vi "PieChart-New.vi"(6 "InitializationValue-Input":T2, 7 "Plot Cluster":T1, 8 "error in (no error)":errorcluster, 9 "Graph Refference's":T3, 10 "Zen Analytics in":refnum<class "Zen Analytics.lvclass">, 11 "Input_Data":dbl[][](array[numeric])=[[1.0, 2.0, 3.0, 4.0, 5.0, 6.0, 7.0, 8.0, 9.0, 10.0], [1.0, 2.0, 3.0, 4.0, 5.0, 6.0, 7.0, 8.0, 9.0, 10.0], [1.0, 2.0, 3.0, 4.0, 5.0, 6.0, 7.0, 8.0, 9.0, 10.0], [1.0, 2.0, 3.0, 4.0, 5.0, 6.0, 7.0, 8.0, 9.0, 10.0], [1.0, 2.0, 3.0, 4.0, 5.0, 6.0, 7.0, 8.0, 9.0, 10.0], [1.0, 2.0, 3.0, 4.0, 5.0, 6.0, 7.0, 8.0, 9.0, 10.0], [1.0, 2.0, 3.0, 4.0, 5.0, 6.0, 7.0, 8.0, 9.0, 10.0], [1.0, 2.0, 3.0, 4.0, 5.0, 6.0, 7.0, 8.0, 9.0, 10.0], [1.0, 2.0, 3.0, 4.0, 6.0, 6.0, 7.0, 8.0, 9.0, 10.0], [1.0, 2.0, 3.0, 4.0, 5.0, 6.0, 7.0, 8.0, 9.0, 10.0]]) -> (0 "error out":errorcluster, 4 "InitializationValues-Output":T2)   [LabVIEW 2019, in "Zen Analytics.lvlib" / "Zen Analytics.lvclass"]
uses:
  Zen Analytics.lvclass
  Dependency/GraphReff.ctl
  Dependency/Plot Cluster.ctl
panel:
  in  "ColorForProduction":u32[](array[colorbox])=[30476, 12845604]
  in  "ColorsForDefects":u32[](array[colorbox])=[10387, 14090395, 38587, 9764938, 14009600, 9961367, 16618491, 12294549, 16752640, 9614336, 35148, 16961, 2228, 13369599, 16740764, 12293546, 8152202, 7498315, 8229484, 8692651, 16744793, 12713794, 32960, 9005056, 7536640, 1638515, 3604546, 13107307, 16734575, 13107258, 4793150, 4934514]
types:
  T1 = typedef "Zen Analytics.lvlib/Zen Analytics.lvclass/Plot Cluster.ctl" = cluster{"Reduced 2D":dbl[][], "Start Index":i32, "No Of New Termnals":i32, "Top/Bottom":bool, "Values Inserted":i32, "Re-Initialised":bool, "Statistical params":string[][], "MeasurementInitializationData":cluster{"Measurement-ID":i32[], "Measurement Names":string[], "NominalValues":dbl[], "LSL":dbl[], "USL":dbl[], "LCL":dbl[], "UCL":dbl[]}, "MeasurementData":cluster{"Measurement ID":i32, "Measurement Name":string, "Nominal Values":dbl, "LSL":dbl, "USL":dbl, "LCL":dbl, "UCL":dbl}[], "ResultData2D":dbl[][], "PlotParameters":cluster{"Trend":cluster{"TrendPlotID":dbl, "PlotProperties":cluster{"FontName":string, "FontSize":dbl, "FontColor":string, "IsBold":bool, "IsItalic":bool, "PlotColor":string}}[], "Histogram":cluster{"HistogramPlotID":dbl, "PlotProperties":cluster{"FontName":string, "FontSize":dbl, "FontColor":string, "IsBold":bool, "IsItalic":bool, "PlotColor":string}}[], "BarPlot":cluster{"BarPlotID":dbl, "BarValuesID":dbl, "PlotProperties":cluster{"FontName":string, "FontSize":dbl, "IsBold":bool, "IsItalic":bool, "FontColor":string}, "Sectors":string[]}[], "PieChart":cluster{"PieChartID":dbl, "PieChartValueID":dbl, "PlotProperties":cluster{"FontName":string, "FontSize":dbl, "IsBold":bool, "IsItalic":bool, "FontColor":string}, "Sectors":string[]}[]}}
  T2 = cluster{"InitializationDefect":dbl[], "InitializationProduction":dbl[]}
  T3 = typedef "Zen Analytics.lvlib/Zen Analytics.lvclass/GraphReff.ctl" = cluster{"HistgramGraph-reff":refnum<vi>[], "BarGraph-reff":refnum<vi>[], "PieGraph-reff":refnum<vi>[], "Lable-reff":refnum<vi>[], "TrendGraph-reff":refnum<vi>[], "CpCpkTable":refnum<vi>}
  T4 = cluster{"PieChartID":dbl, "PieChartValueID":dbl, "PlotProperties":cluster{"FontName":string, "FontSize":dbl, "IsBold":bool, "IsItalic":bool, "FontColor":string}, "Sectors":string[]}[]
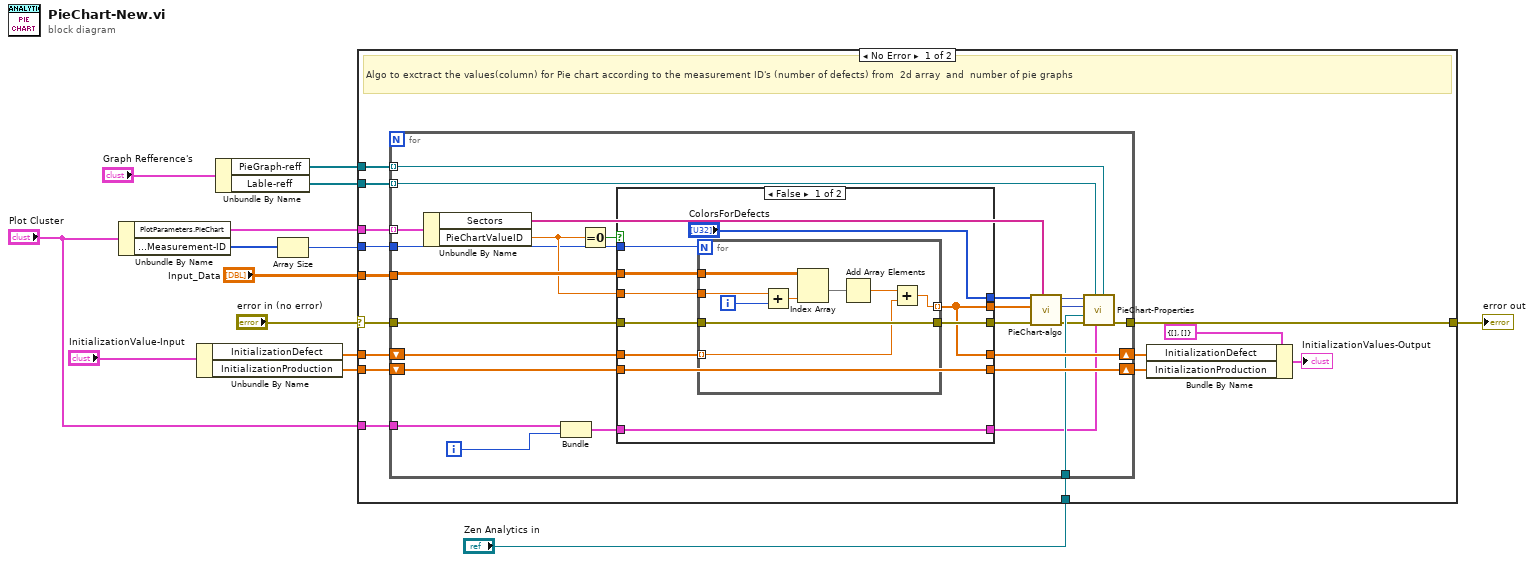
[diagram p0: block diagram]
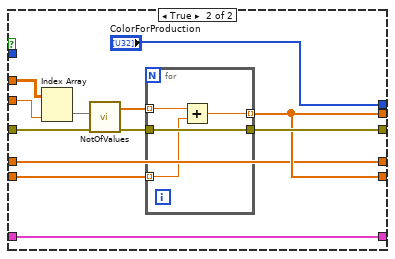
[diagram p2: hidden frame]
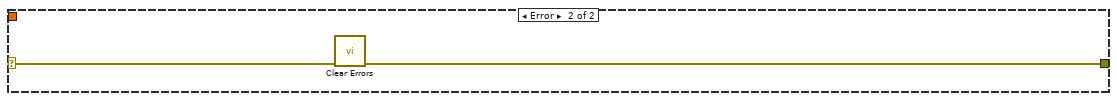
[diagram p3: hidden frame]
diagram:
  n1 = Unbundle By Name("Plot Cluster") -> ("PlotParameters.PieChart"=w7:T4, "MeasurementInitializationData.Measurement-ID"=w2:i32[])
  n2 = Unbundle By Name("InitializationValue-Input") -> ("InitializationDefect"=w8:dbl[], "InitializationProduction"=w9:dbl[])
  n3 = Unbundle By Name("Graph Refference's") -> ("PieGraph-reff"=w13:refnum<vi>[], "Lable-reff"=w11:refnum<vi>[])
  n4 = Array Size(array=w2) -> (size(s)=w1:i32)
  n5 = case shown="No Error" "error in (no error)" {
    selector: "error in (no error)" -> [w27 w91]
    tunnel: [w28 w90] -> w4
    tunnel: w13 -> [w26 _]
    tunnel: w7 -> [w29 _]
    tunnel: "Input_Data" -> [w25 _]
    tunnel: w11 -> [w24 _]
    tunnel: w9 -> [w23 _]
    tunnel: w8 -> [w22 _]
    tunnel: "Plot Cluster" -> [w17 _]
    tunnel: "Zen Analytics in" -> [w16 _]
    tunnel: w1 -> [w15 _]
    frame No Error {
      # "Algo to exctract the values(column) for Pie chart according to the measurement ID's (number of defects) from  2d array  and  number of pie graphs"
      n6 = for {
        tunnel: w29 -> [w43] mode=indexing
        tunnel: [w54] -> w28
        tunnel: w27 -> [w53]
        tunnel: w26 -> [w52] mode=indexing
        tunnel: w25 -> [w51]
        tunnel: w24 -> [w50] mode=indexing
        shift-right: [w48] -> w18
        shift-left: w23 -> [w49]
        shift-right: [w46] -> w19
        shift-left: w22 -> [w47]
        tunnel: w17 -> [w45]
        tunnel: w16 -> [w41]
        tunnel: w15 -> [w31]
        i -> [w42]
        n7 = Unbundle By Name(w43) -> ("Sectors"=w30:string[], "PieChartValueID"=w32:dbl)
        n8 = Bundle("Plot Cluster"=w45, w42) -> (w44:cluster{"Plot Cluster":T1, i32})  [unwired: 1 in]
        n9 = Equal To 0?(x=w32) -> (x = 0?=w40:bool)
        n10 = case shown="False" w40 {
          tunnel: w51 -> [w64 w84]
          tunnel: w53 -> [w62 w85]
          tunnel: [w63 w80] -> w39
          tunnel: [w58 w77] -> w38
          tunnel: w31 -> [w55 _]
          tunnel: w32 -> [w61 w83]
          tunnel: ["ColorsForDefects" "ColorForProduction"] -> w37
          tunnel: w49 -> [w60 w78]
          tunnel: [w60 w77] -> w48
          tunnel: w47 -> [w59 w76]
          tunnel: [w58 w76] -> w46
          tunnel: w44 -> [w56 w74]
          tunnel: [w56 w74] -> w33
          frame False {
            n11 = for {
              N: w55 -> [_]
              tunnel: w64 -> [w73]
              tunnel: [w67] -> w58 mode=indexing
              tunnel: [w69] -> w63
              tunnel: w62 -> [w69]
              tunnel: w61 -> [w68]
              tunnel: w59 -> [w65] mode=indexing
              i -> [w71]
              n12 = Add(x=w68, y=w71) -> (x+y=w72:dbl)
              n13 = Index Array(array=w73, index (col)=w72) -> (element=w70:dbl[])  [unwired: 1 in]
              n14 = Add Array Elements(numeric array=w70) -> (sum=w66:dbl)
              n15 = Add(x=w66, y=w65) -> (x+y=w67:dbl)
            }
          }
          frame True {
            n16 = Index Array(array=w84, index (col)=w83) -> (element=w82:dbl[])  [unwired: 1 in]
            n17 = call "NotOfValues.vi"("error in (no error)"=w85, "Inputdata"=w82) -> ("error out"=w81:errorcluster, "Outputvalues"=w79:dbl[])  [unwired: 8 in]
            n18 = for {
              tunnel: w79 -> [w87] mode=indexing
              tunnel: [w89] -> w77 mode=indexing
              tunnel: w81 -> [w88]
              tunnel: [w88] -> w80
              tunnel: w78 -> [w86] mode=indexing
              n19 = Add(x=w87, y=w86) -> (x+y=w89:dbl)
            }
          }
        }
        n20 = call "PieChart-algo.vi"("Defect Names"=w30, "error in (no error)"=w39, "Array Of Values"=w38, "Colors"=w37) -> ("error out"=w35:errorcluster, "Lable"=w36:picture, "Pie"=w34:picture)  [unwired: 5 in]
        n21 = call "PieChart-Properties.vi"("Yeild-chart 2"=w52, "Plot Cluster Index out"=w33, "Label Total"=w50, "error in (no error)"=w35, "Zen Analytics in"=w41, "Lable"=w36, "YeildChart"=w34) -> ("error out"=w54:errorcluster)  [unwired: 4 in]
      }
      n22 = Bundle By Name(cluster=T2 {"InitializationDefect"=[], "InitializationProduction"=[]} ("InitializationValues-Output"), "InitializationDefect"=w19, "InitializationProduction"=w18) -> (→"InitializationValues-Output":T2)
    }
    frame Error {
      n23 = call <vilib>:"Clear Errors.vi"("error in (no error)"=w91) -> ("error out"=w90:errorcluster)  [unwired: 5 in, 1 out]
    }
  }
  "error out" <- w4
